vi "checkbox_init.vi"(0 "MulticolumnListbox in":refnum<vi>, 5 "labels":string[](array[string]), 7 "heat inputs":tag[](array[tag]), 9 "heat outputs":refnum<k21>[](array[refnum]), 11 "mag inputs":tag[](array[tag])) -> (4 "MulticolumnListbox out":refnum<vi>, 6 "checkbox array":i32[](array[numeric]), 10 "i/o array":T1(array[cluster]))   [LabVIEW 2015]
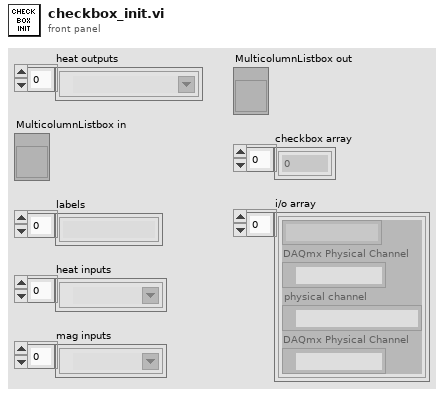
[diagram p1: front panel]
types:
  T1 = cluster{string, "DAQmx Physical Channel":tag, "physical channel":refnum<k21>, "DAQmx Physical Channel":tag}[]
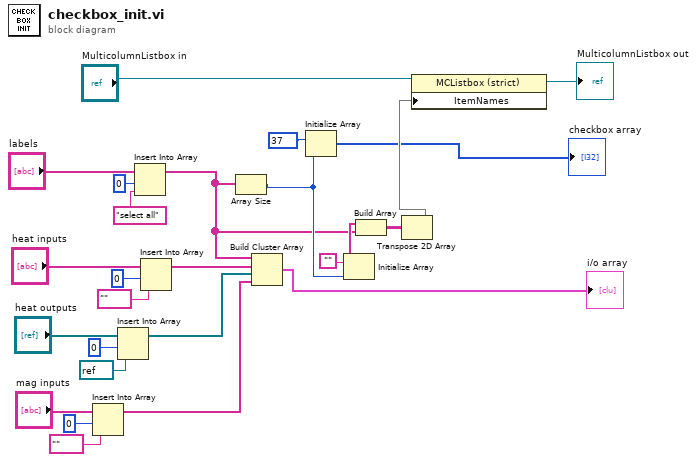
[diagram p0: block diagram]
diagram:
  n1 = Insert Into Array(array="mag inputs", index=0, new element=tag "" ("new element/subarray")) -> (w11:tag[])
  n2 = Insert Into Array(array="heat outputs", index=0, new element=refnum<k21> refnum ("new element/subarray")) -> (w6:refnum<k21>[])
  n3 = Insert Into Array(array="labels", index=0, new element="select all" ("new element/subarray")) -> (w13:string[])
  n4 = Insert Into Array(array="heat inputs", index=0, new element=tag "" ("new element/subarray")) -> (w1:tag[])
  n5 = Array Size(array=w13) -> (size(s)=w17:i32)
  n6 = Build Cluster Array(w13, w1, w6, w11) -> (→"i/o array":T1)
  n7 = Initialize Array(37, w17) -> (→"checkbox array":i32[])
  n8 = Initialize Array("", w17) -> (w20:string[])
  n9 = Build Array(w20, w13) -> (w21:string[][])
  n10 = Transpose 2D Array(2D array=w21) -> (transposed array=w23:string[][])
  n11 = property on="Property Node" class="MCListbox (strict)"(reference="MulticolumnListbox in", "ItemNames"=w23) -> (reference out=→"MulticolumnListbox out":refnum<vi>)  [unwired: 1 in, 1 out]
